vi "test_CCDGetConfig.vi"(6 "Delay between send and receive [ms]":i32=100, 7 "Test should pass":bool=TRUE, 8 "error in":errorcluster, 9 "tear down connection":bool=TRUE, 10 "set-up a connection":bool=TRUE, 11 "device selection":enum16{"monochromator", "CCD", "SCD"}(ring)=enum."CCD") -> (0 "error out":errorcluster)   [LabVIEW 2023]
uses:
  <vilib>/addons/_JKI Toolkits/Caraya/classes/Test/Test.lvclass
  <vilib>/addons/_JKI Toolkits/Caraya/classes/Assert/Assert.lvclass
  Classes/CCD/CCD.lvclass
  Classes/CCD/Gain.ctl
  Classes/CCD/Type.ctl
  Classes/CCD/Event.ctl
  Classes/CCD/Signal.ctl
  Classes/CCD/Speed.ctl
  Classes/CCD/Trigger.ctl
  Classes/CCD/GetConfig.ctl
  <vilib>/addons/_JKI Toolkits/Caraya/classes/Assert/Assert Not Error.vi
  <vilib>/addons/_JKI Toolkits/Caraya/classes/Assert/Assert Equal Value_Variant.vi
  Classes/CCD/SupportedFeatures.ctl
panel:
  out "config-text pairs":string[][](array[string])
  out "config-JSON pairs":string[][](array[string])
  out "config-JSON string":string="{\"configuration\":{\"CenterWavelength\":0,\"ChipHSpacing\":\"260\",\"ChipHeight\":\"256\",\"ChipName\":\"CCD30-11-1-275\",\"ChipSerialNumber\":\"20091-22-21\",\"ChipVSpacing\":\"260\",\"ChipWidth\":\"1024\",\"DeviceType\":\"HORIBA Scientific Syncerity\",\"FitParameters\":[0,1,0,0,0],\"Gains\":[{\"Info\":\"Best Dynamic Range\",\"Token\":1},{\"Info\":\"High Light\",\"Token\":0},{\"Info\":\"High Sensitivity\",\"Token\":2}],\"HardwareAvgAvailable\":\"False\",\"LineScan\":\"False\",\"ProductId\":\"13\",\"SerialNumber\":\"Camera SN:  2244\",\"Signals\":[{\"Events\":[{\"Name\":\"Ready For Trigger\",\"Token\":1,\"Types\":[{\"Name\":\"TTL Active Low\",\"Token\":1},{\"Name\":\"TTL Active High\",\"Token\":0}]},{\"Name\":\"Shutter Open\",\"Token\":3,\"Types\":[{\"Name\":\"TTL Active Low\",\"Token\":1},{\"Name\":\"TTL Active High\",\"Token\":0}]},{\"Name\":\"Start Experiment\",\"Token\":0,\"Types\":[{\"Name\":\"TTL Active Low\",\"Token\":1},{\"Name\":\"TTL Active High\",\"Token\":0}]},{\"Name\":\"Reserved-DO NOT USE\",\"Token\":2,\"Types\":[{\"Name\":\"TTL Active Low\",\"Token\":1},{\"Name\":\"TTL Active High\",\"Token\":0}]}],\"Name\":\"Signal Output\",\"Token\":0}],\"Speeds\":[{\"Info\":\" 1 MHz       \",\"Token\":1},{\"Info\":\"45 kHz       \",\"Token\":0},{\"Info\":\"500 kHz Wrap\",\"Token\":127},{\"Info\":\" 1 MHz Ultra \",\"Token\":2}],\"SupportedFeatures\":{\"CF_3PositionSlit\":\"False\",\"CF_CMOSOffsetCorrection\":\"False\",\"CF_Cleaning\":\"True\",\"CF_DSP\":\"False\",\"CF_DSPBin2X\":\"False\",\"CF_DelayAfterTrigger\":\"False\",\"CF_Delays\":\"False\",\"CF_EMCCD\":\"False\",\"CF_EShutter\":\"False\",\"CF_HDR\":\"False\",\"CF_Image\":\"True\",\"CF_MemorySlots\":\"True\",\"CF_Metadata\":\"False\",\"CF_MultipleExposeTimes\":\"False\",\"CF_MultipleSensors\":\"False\",\"CF_PulseSummation\":\"False\",\"CF_ROIs\":\"True\",\"CF_Signals\":\"True\",\"CF_Spectra\":\"True\",\"CF_TriggerQualifier\":\"False\",\"CF_Triggers\":\"True\"},\"Triggers\":[{\"Events\":[{\"Name\":\"Each - For Each Acq\",\"Token\":1,\"Types\":[{\"Name\":\"TTL Rising  Edge\",\"Token\":1},{\"Name\":\"TTL Falling Edge\",\"Token\":0}]},{\"Name\":\"Once - Start All\",\"Token\":0,\"Types\":[{\"Name\":\"TTL Rising  Edge\",\"Token\":1},{\"Name\":\"TTL Falling Edge\",\"Token\":0}]}],\"Name\":\"Trigger Input\",\"Token\":0}],\"Version\":\"Syncerity Ver 1.001.7.1\"}}"
  # "Connector Pane"
  # "Locals"
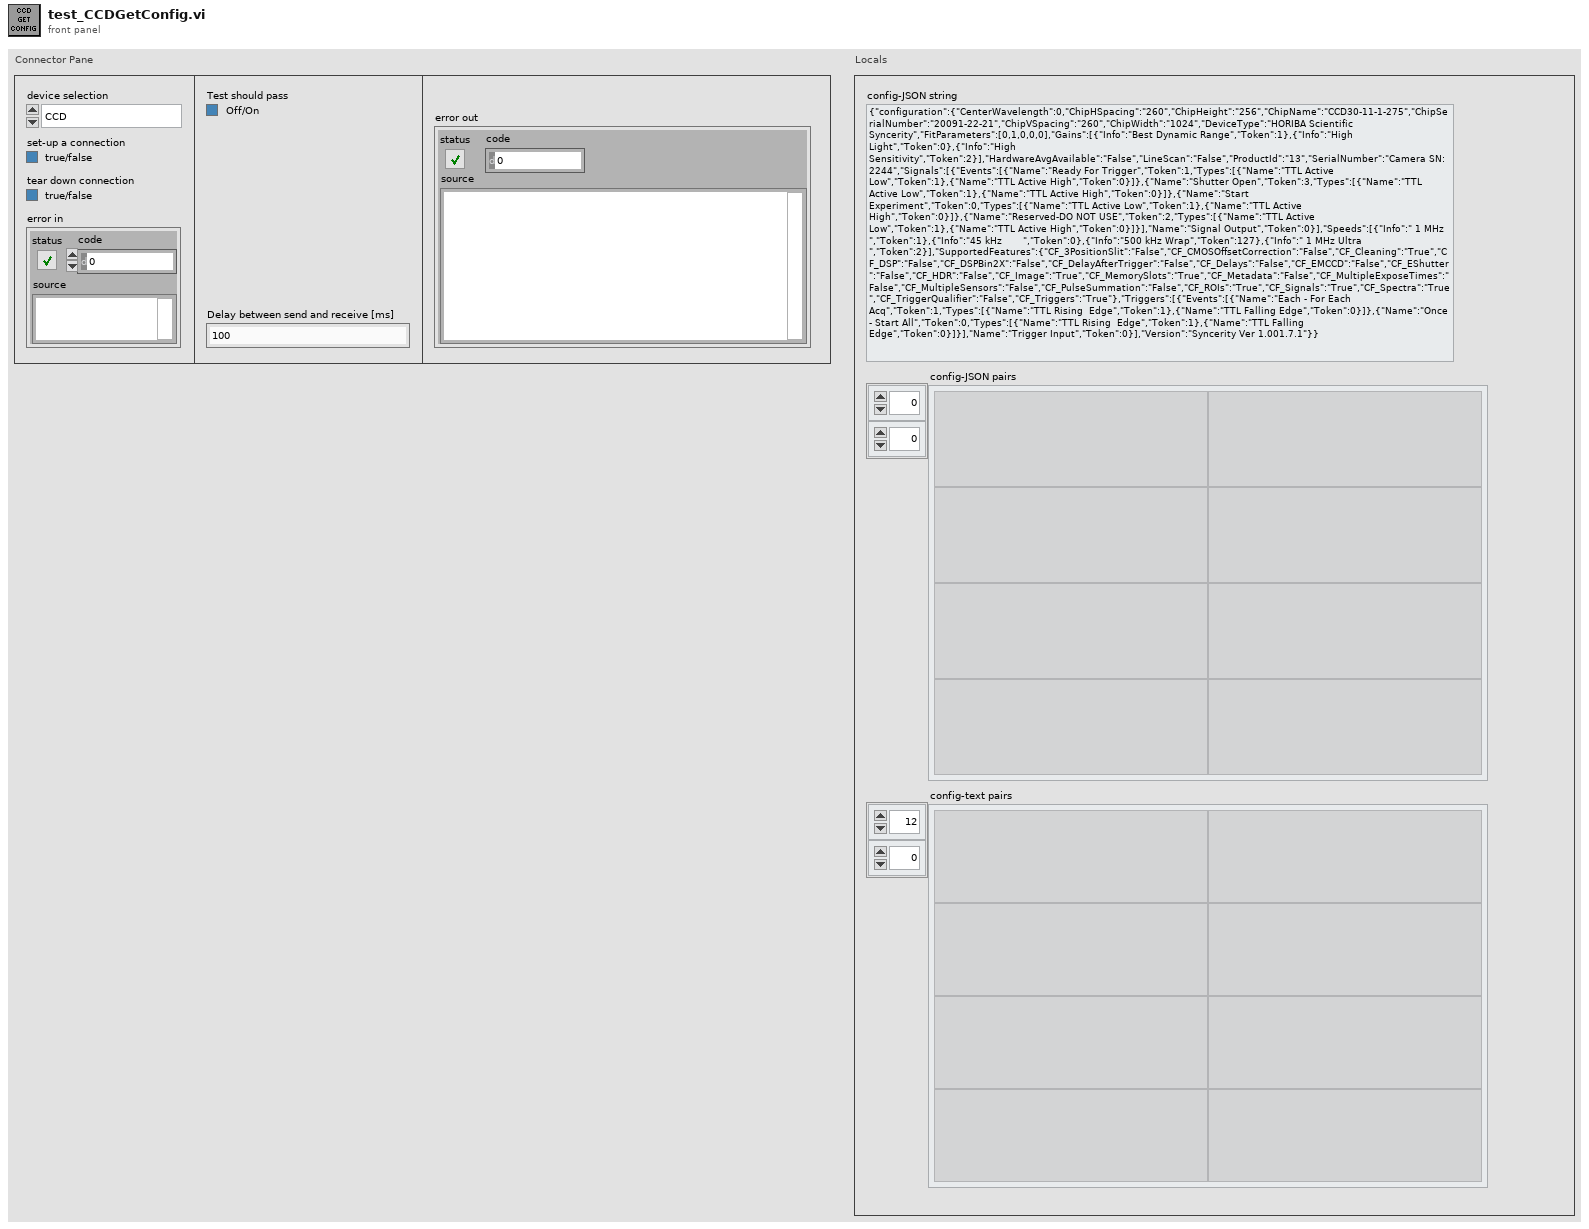
[diagram p1: front panel]
types:
  T1 = typedef "CCD.lvclass/GetConfig.ctl" = cluster{"centerWavelength":dbl, "chipHSpacing":dbl, "chipHeight":dbl, "chipName":string, "chipSerialNumber":string, "chipVSpacing":dbl, "chipWidth":dbl, "deviceType":string, "fitParameters":dbl[], "gains":T2[], "hardwareAvgAvailable":bool, "lineScan":bool, "productId":string, "serialNumber":string, "signals":T3[], "speeds":T6[], "supportedFeatures":T7, "triggers":T8[], "version":string}
  T2 = typedef "CCD.lvclass/Gain.ctl" = cluster{"info":string, "token":i32}
  T3 = typedef "CCD.lvclass/Signal.ctl" = cluster{"events":T4[], "name":string, "token":i32}
  T4 = typedef "CCD.lvclass/Event.ctl" = cluster{"name":string, "token":i32, "types":T5[]}
  T5 = typedef "CCD.lvclass/Type.ctl" = cluster{"name":string, "token":i32}
  T6 = typedef "CCD.lvclass/Speed.ctl" = cluster{"info":string, "token":i32}
  T7 = typedef "CCD.lvclass/SupportedFeatures.ctl" = cluster{"cf_3PositionSlit":bool, "cf_CMOSOffsetCorrection":bool, "cf_Cleaning":bool, "cf_DSP":bool, "cf_DSPBin2X":bool, "cf_DelayAfterTrigger":bool, "cf_Delays":bool, "cf_EMCCD":bool, "cf_EShutter":bool, "cf_HDR":bool, "cf_Image":bool, "cf_MemorySlots":bool, "cf_Metadata":bool, "cf_MultipleExposeTimes":bool, "cf_MultipleSensors":bool, "cf_PulseSummation":bool, "cf_ROIs":bool, "cf_Signals":bool, "cf_Spectra":bool, "cf_TriggerQualifier":bool, "cf_Triggers":bool}
  T8 = typedef "CCD.lvclass/Trigger.ctl" = cluster{"events":T4[], "name":string, "token":i32}
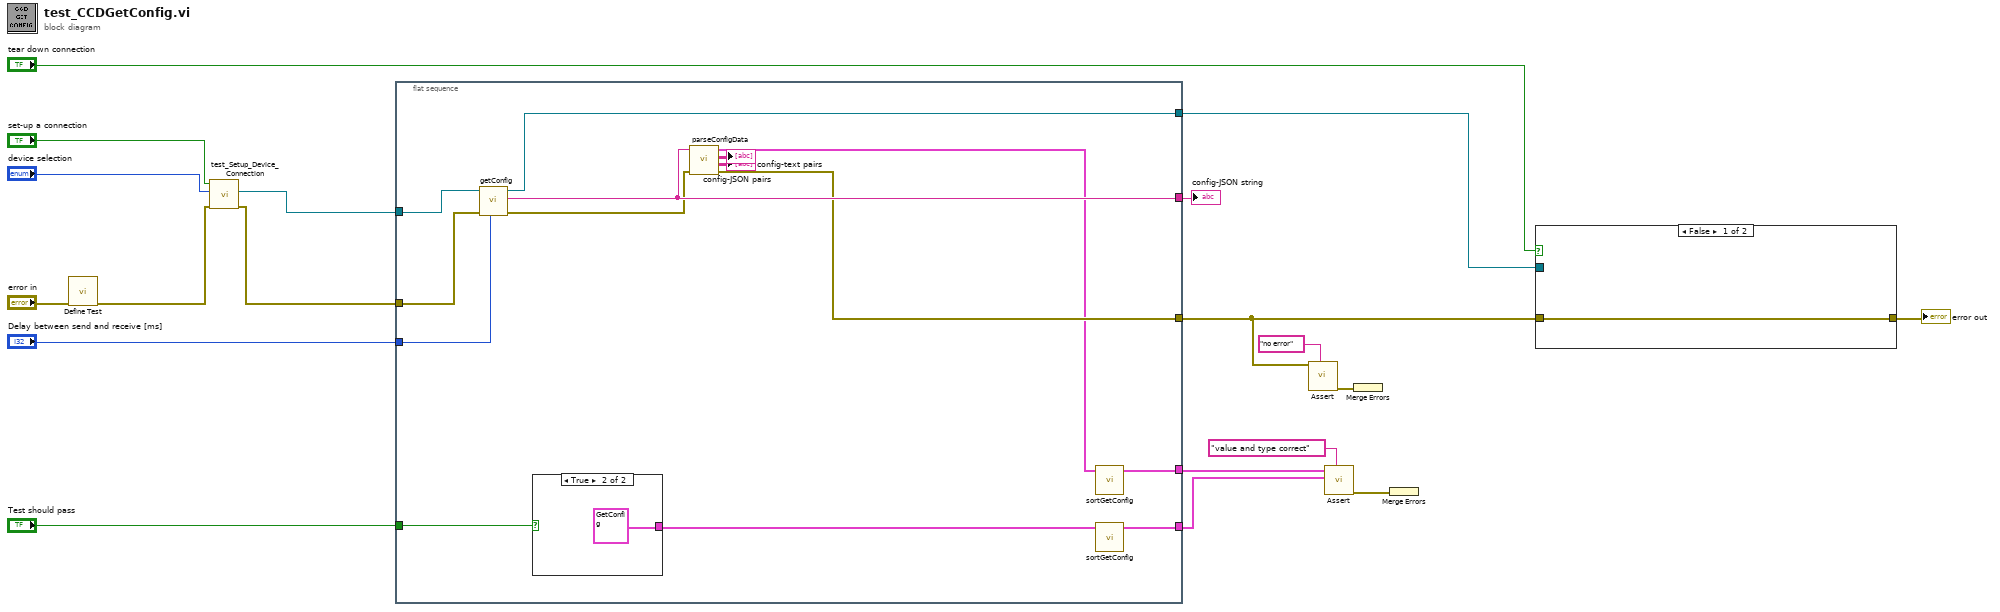
[diagram p0: block diagram]
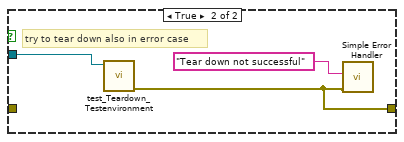
[diagram p3: hidden frame]
diagram:
  n1 = call <vilib>:"Define Test.vi"("error in (no error)"="error in") -> ("error out"=w6:errorcluster)  [unwired: 9 in, 1 out]
  n2 = call "test_Setup_Device_Connection.vi"("error in (no error)"=w6, "device selection"="device selection", "set-up a connection"="set-up a connection") -> ("error out"=w4:errorcluster, "CCD.lvclass"=w5:refnum<class "CCD.lvclass">)  [unwired: 5 in, 2 out]
  n3 = flat-sequence {
    tunnel: [w28] -> w17
    tunnel: w4 -> [w33]
    tunnel: w5 -> [w32]
    tunnel: [w26] -> w11
    tunnel: "Test should pass" -> [w31]
    tunnel: [w30] -> w10
    tunnel: "Delay between send and receive [ms]" -> [w29]
    tunnel: [w22] -> w2
    tunnel: [w20] -> w1
    frame #0 {
      n4 = call "getConfig.vi"("Delay between send and receive [ms]"=w29, "error in (no error)"=w33, "CCD in"=w32) -> ("error out"=w27:errorcluster, "config-JSON string"=w28:string, "CCD out"=w30:refnum<class "CCD.lvclass">)  [unwired: 6 in]
      n5 = case shown="True" w31 {
        tunnel: [_ T1 {"centerWavelength"=0.0, "chipHSpacing"=260.0, "chipHeight"=256.0, "chipName"="CCD30-11-1-275", "chipSerialNumber"="20091-22-21", "chipVSpacing"=260.0, "chipWidth"=1024.0, "deviceType"="HORIBA Scientific Syncerity", "fitParameters"=[0.0, 1.0, 0.0, 0.0, 0.0], "gains"=[{"info"="Best Dynamic Range", "token"=1}, {"info"="High Sensitivity", "token"=2}, {"info"="High Light", "token"=0}], "hardwareAvgAvailable"=FALSE, "lineScan"=FALSE, "productId"="13", "serialNumber"="Camera SN:  2244", "signals"=[{"events"=[{"name"="Ready For Trigger", "token"=1, "types"=[{"name"="TTL Active Low", "token"=1}, {"name"="TTL Active High", "token"=0}]}, {"name"="Shutter Open", "token"=3, "types"=[{"name"="TTL Active Low", "token"=1}, {"name"="TTL Active High", "token"=0}]}, {"name"="Reserved-DO NOT USE", "token"=2, "types"=[{"name"="TTL Active Low", "token"=1}, {"name"="TTL Active High", "token"=0}]}, {"name"="Start Experiment", "token"=0, "types"=[{"name"="TTL Active Low", "token"=1}, {"name"="TTL Active High", "token"=0}]}], "name"="Signal Output", "token"=0}], "speeds"=[{"info"=" 1 MHz       ", "token"=1}, {"info"="500 kHz Wrap", "token"=127}, {"info"=" 1 MHz Ultra ", "token"=2}, {"info"="45 kHz       ", "token"=0}], "supportedFeatures"={"cf_3PositionSlit"=FALSE, "cf_CMOSOffsetCorrection"=FALSE, "cf_Cleaning"=TRUE, "cf_DSP"=FALSE, "cf_DSPBin2X"=FALSE, "cf_DelayAfterTrigger"=FALSE, "cf_Delays"=FALSE, "cf_EMCCD"=FALSE, "cf_EShutter"=FALSE, "cf_HDR"=FALSE, "cf_Image"=TRUE, "cf_MemorySlots"=TRUE, "cf_Metadata"=FALSE, "cf_MultipleExposeTimes"=FALSE, "cf_MultipleSensors"=FALSE, "cf_PulseSummation"=FALSE, "cf_ROIs"=TRUE, "cf_Signals"=TRUE, "cf_Spectra"=TRUE, "cf_TriggerQualifier"=FALSE, "cf_Triggers"=TRUE}, "triggers"=[{"events"=[{"name"="Each - For Each Acq", "token"=1, "types"=[{"name"="TTL Rising  Edge", "token"=1}, {"name"="TTL Falling Edge", "token"=0}]}, {"name"="Once - Start All", "token"=0, "types"=[{"name"="TTL Rising  Edge", "token"=1}, {"name"="TTL Falling Edge", "token"=0}]}], "name"="Trigger Input", "token"=0}], "version"="Syncerity Ver 1.001.7.1"} ("config data 2")] -> w21
        frame False {
        }
        frame True {
        }
      }
      n6 = call "parseConfigData.vi"("error in (no error)"=w27, "results-JSON string"=w28) -> ("error out"=w26:errorcluster, "config-text pairs"=→"config-text pairs":string[][], "config-JSON pairs"=→"config-JSON pairs":string[][], "config data"=w23:T1)  [unwired: 6 in]
      n7 = call "sortGetConfig.vi"("config data in"=w23) -> ("config data out"=w22:T1)  [unwired: 10 in]
      n8 = call "sortGetConfig.vi"("config data in"=w21) -> ("config data out"=w20:T1)  [unwired: 10 in]
    }
  }
  n9 = call-poly <vilib>:"Assert.vi"("Label"="no error" ("Label (VI Title)"), "Not Error?"=w11) -> ("error out"=w13:errorcluster)  [unwired: 8 in, 1 out]
  n10 = call-poly <vilib>:"Assert.vi"("Label"="value and type correct" ("Label (VI Title)"), "Y"=w1, "X"=w2) -> ("error out"=w18:errorcluster)  [unwired: 7 in, 1 out]
  n11 = Merge Errors(w13) -> ()  [unwired: 1 out]
  n12 = Merge Errors(w18) -> ()  [unwired: 1 out]
  n13 = case shown="False" "tear down connection" {
    tunnel: w10 -> [_ w37]
    tunnel: [w35 w36] -> w9
    tunnel: w11 -> [w35 _]
    frame False {
    }
    frame True {
      # "try to tear down also in error case"
      n14 = call "test_Teardown_Testenvironment.vi"("GenericDevice.lvclass"=w37) -> ("error out"=w36:errorcluster)  [unwired: 9 in, 1 out]
      n15 = call <vilib>:"Simple Error Handler.vi"("error source (\" \")"="Tear down not successful" ("error source (\" \")"), "error in (no error)"=w36) -> ()  [unwired: 3 in, 5 out]
    }
  }
  "error out" <- w9
  "config-JSON string" <- w17
